vi "Point and Shoot Bias.vi"(8 "Error in (no error)":errorcluster, 11 "Cluster":cluster{"Initial x":dbl, "Initial y":dbl}) -> (0 "error out":errorcluster, 3 "output cluster":cluster{"Initial x":dbl, "Initial y":dbl})   [LabVIEW 2025]
uses:
  <userlib>/Nanonis Prog Interface V5e/Nanonis Prog Interface.lvlib
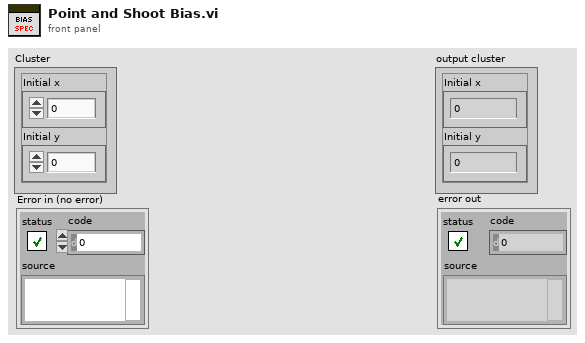
[diagram p1: front panel]
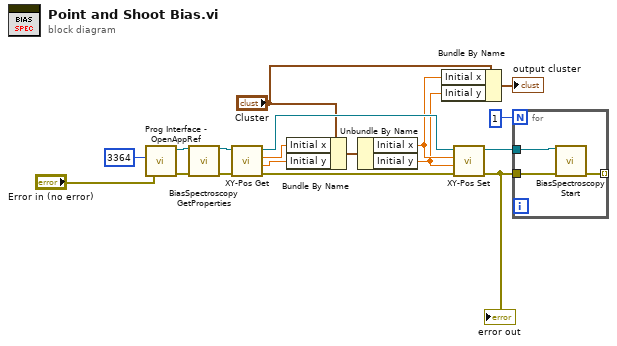
[diagram p0: block diagram]
diagram:
  n1 = call <userlib>:"Prog Interface - OpenAppRef.vi"("Error in (no error)"="Error in (no error)", "Port number (3364)"=u32 3364) -> ("Error out"=w17:errorcluster, "Application reference"=w18:refnum<vi>)  [unwired: 4 in]
  n2 = call <userlib>:"BiasSpectroscopy GetProperties.vi"("Application ref in"=w18, "Error in (no error)"=w17) -> ("Application ref out"=w13:refnum<vi>, "Error out"=w14:errorcluster)  [unwired: 6 in, 6 out]
  n3 = call <userlib>:"XY-Pos Get.vi"("error in (no error)"=w14, "Application ref in"=w13) -> ("error out"=w16:errorcluster, "Y (m)"=w7:sgl, "X (m)"=w8:sgl, "Application ref out"=w15:refnum<vi>)  [unwired: 5 in]
  n4 = Bundle By Name(cluster="Cluster", "Initial x"=w8, "Initial y"=w7) -> (w6:cluster{"Initial x":dbl, "Initial y":dbl})
  n5 = Unbundle By Name(w6) -> ("Initial x"=w4:dbl, "Initial y"=w3:dbl)
  n6 = Bundle By Name(cluster="Cluster", "Initial x"=w4, "Initial y"=w3) -> (→"output cluster":cluster{"Initial x":dbl, "Initial y":dbl})
  n7 = call <userlib>:"XY-Pos Set.vi"("error in (no error)"=w16, "Y (m)"=w3, "X (m)"=w4, "Application ref in"=w15) -> ("error out"=w10:errorcluster, "Application ref out"=w11:refnum<vi>)  [unwired: 4 in]
  "error out" <- w10
  n8 = for {
    N: 1 -> [_]
    tunnel: [w21] -> _ mode=indexing
    tunnel: w11 -> [w20]
    tunnel: w10 -> [w19]
    n9 = call <userlib>:"BiasSpectroscopy Start.vi"("Application ref in"=w20, "Error in (no error)"=w19) -> ("Error out"=w21:errorcluster)  [unwired: 9 in, 4 out]
  }
